vi "Set Max Gain.vi"(8 "error in (no error)":errorcluster, 10 "Gain":i32=50 min=0 max=100, 11 "CameraDevRef":T1={"Camera Address"="192.168.0.90", "CameraStatus"={"status"=FALSE, "code"=0, "source"=""}, "Acquire Image Notifier"=refnum}) -> (0 "error out":errorcluster, 3 "CameraDevRef Out":T1)   [LabVIEW 2013]
doc: "Specifies the brightness setting of the camera you specify.\n\nThis software is licensed. Open the labview\\readme\\WPI Robotics Library Open Source License.txt file for more information."
uses:
  <vilib>/Rock Robotics/WPI/Camera/WPI_CameraDevRef.ctl
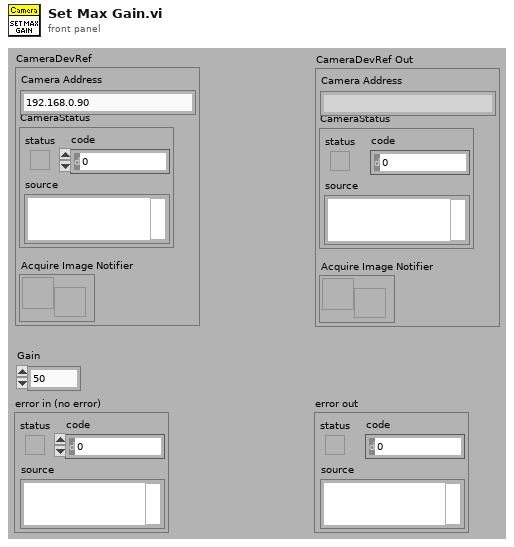
[diagram p1: front panel]
types:
  T1 = typedef "WPI_CameraDevRef.ctl" = cluster{"Camera Address":string, "CameraStatus":errorcluster, "Acquire Image Notifier":refnum<notifier>}
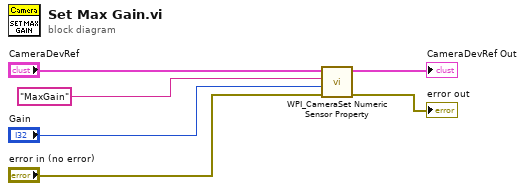
[diagram p0: block diagram]
diagram:
  n1 = call <vilib>:"WPI_CameraSet Numeric Sensor Property.vi"("error in (no error)"="error in (no error)", "Value"="Gain", "Property Name"="MaxGain", "CameraDevRef"="CameraDevRef") -> ("error out"=→"error out":errorcluster, "CameraDevRef out"=→"CameraDevRef Out":T1)  [unwired: 4 in, 2 out]
